vi "Replace Gray.vi"(11 "Image 2":T1) -> (3 "Image":T1(plugin-control))   [LabVIEW 2015]
uses:
  <vilib>/vision/Image Controls.llb/IMAQ Image.ctl
panel:
  out "matrix":u32[][](array[numeric])
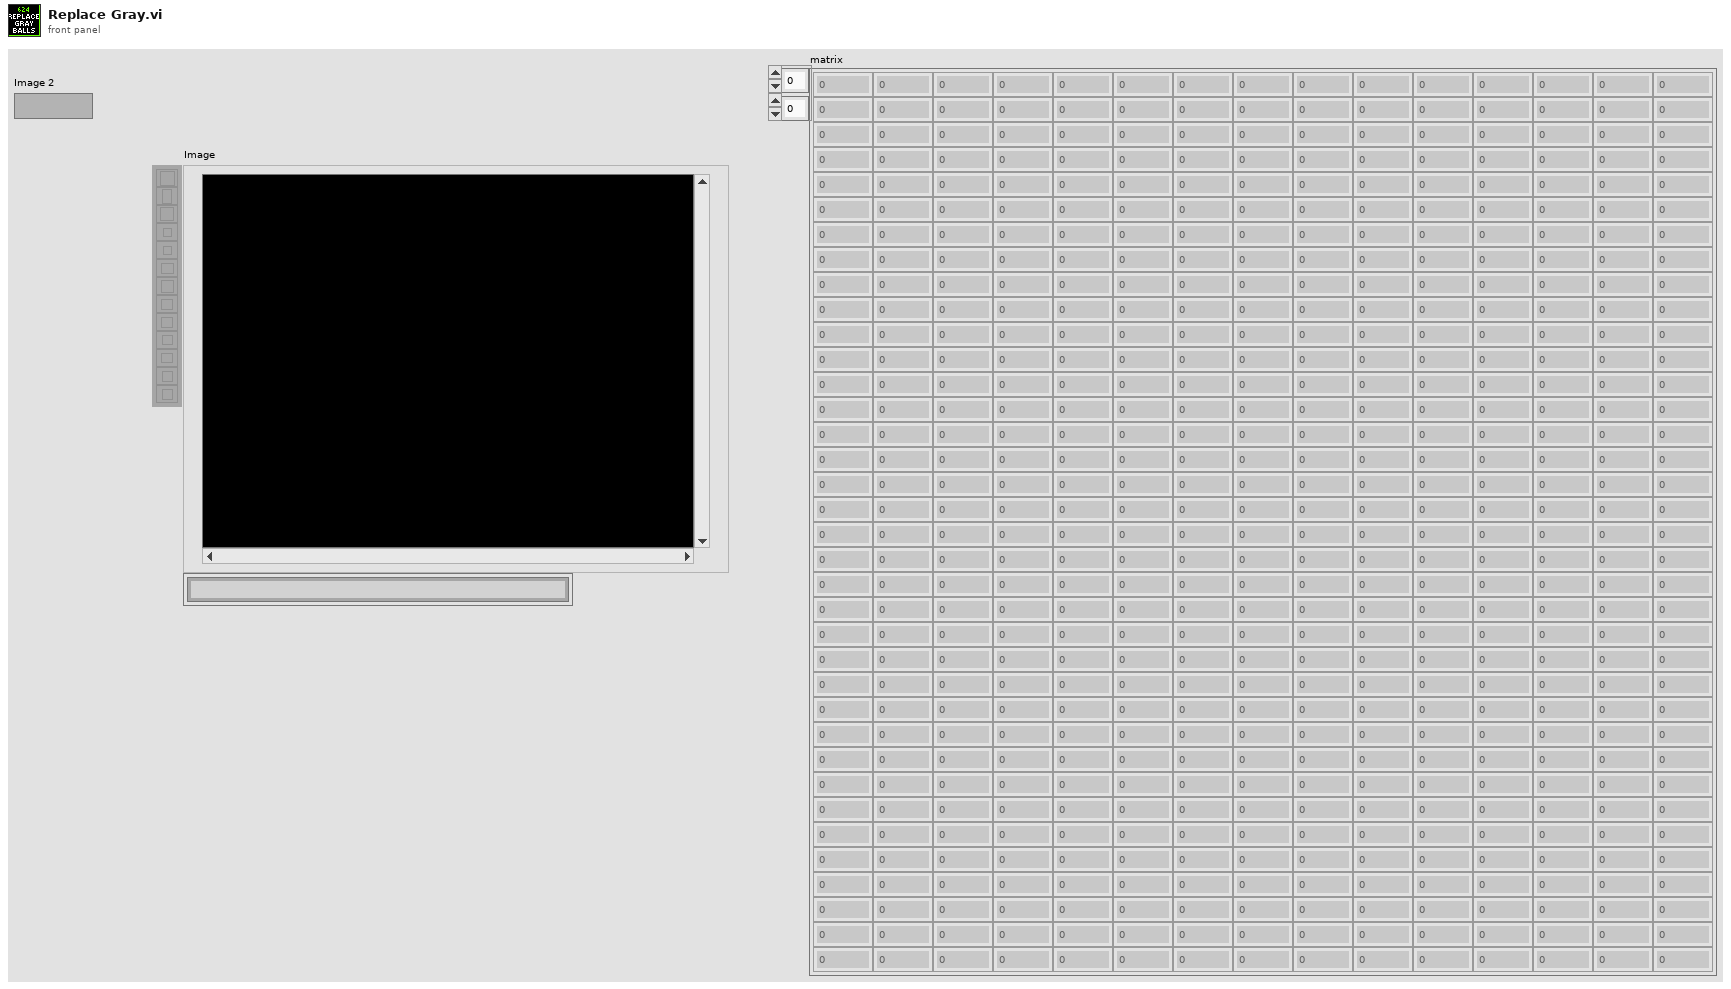
[diagram p1: front panel]
types:
  T1 = typedef "IMAQ Image.ctl" = refnum<image>
  T2 = typedef "Image Type" = u32
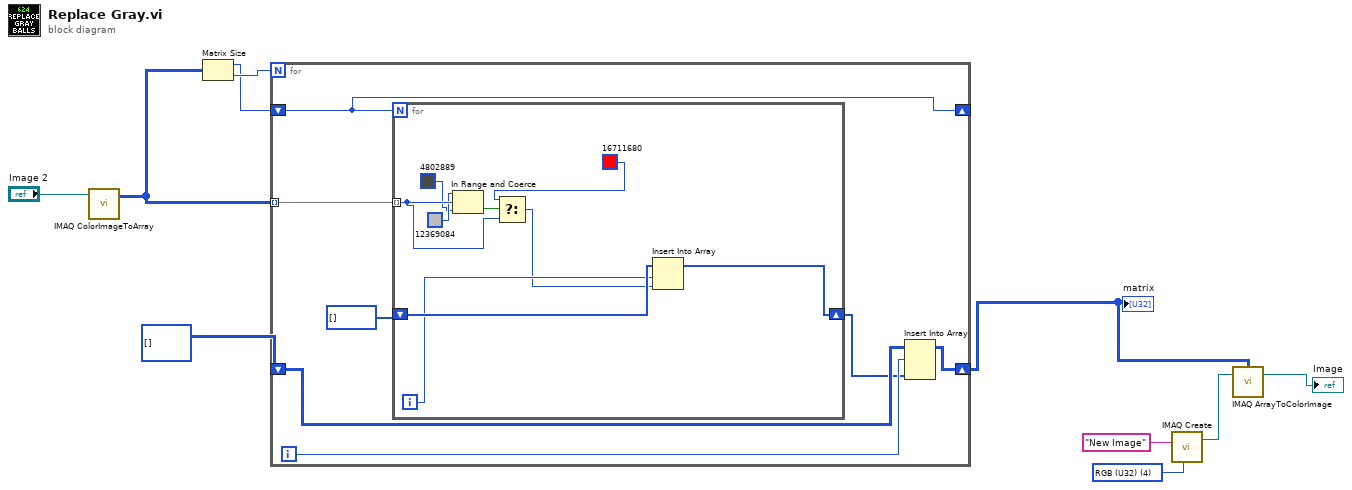
[diagram p0: block diagram]
diagram:
  w4 = T2 4 items=["Grayscale (U8)", "Grayscale (I16)", "Grayscale (SGL)", "Complex (CSG)", "RGB (U32)", "HSL (U32)", "RGB (U64)", "Grayscale (U16)"] ("Image Type")
  n1 = call "IMAQ ColorImageToArray"("Image"="Image 2") -> ("Image Pixels (U32)"=w5:u32[][])  [unwired: 3 in, 2 out]
  n2 = Matrix Size(0:w5) -> (1:w9:i32, 2:w10:i32)
  n3 = for {
    N: w10 -> [_]
    shift-right: [w16] -> w2
    shift-left: u32[][] [] ("matrix") -> [w15]
    shift-right: [w17] -> _
    shift-left: w9 -> [w17]
    tunnel: w5 -> [w14] mode=indexing
    i -> [w13]
    n4 = for {
      N: w17 -> [_]
      shift-right: [w25] -> w11
      shift-left: u32[] [] ("Image Pixels (U32)") -> [w26]
      tunnel: w14 -> [w21] mode=indexing
      i -> [w24]
      n5 = In Range and Coerce(upper limit=u32 12369084, x=w21, lower limit=u32 4802889) -> (In Range?=w20:bool)  [unwired: 1 out]
      n6 = Select(t=u32 16711680, s=w20, f=w21) -> (s? t:f=w23:u32)
      n7 = Insert Into Array(array=w26, index=w24, new element=w23) -> (w25:u32[])
    }
    n8 = Insert Into Array(array=w15, index (row)=w13, new element=w11) -> (w16:u32[][])  [unwired: 1 in]
  }
  "matrix" <- w2
  n9 = call "IMAQ Create"("Image Name"="New Image", "Image Type"=w4) -> ("New Image"=w8:T1)  [unwired: 3 in, 1 out]
  n10 = call "IMAQ ArrayToColorImage"("Image Pixels (U32)"=w2, "Image"=w8) -> ("Image Out"=→"Image":T1)  [unwired: 3 in, 1 out]
